vi "RT Main.vi"() -> ()   [LabVIEW 2016]
doc: "This template is for the Queued Message Handler design pattern.\n\nThe Event Handling Loop generates messages based on user interface actions.\n\nThe Message Handling Loop processes messages generated by the Event Handling Loop, or by other messages. The messages are string values, so new messages can be added easily to the Message Cases case structure in the Message Handling Loop. Each message cluster can also provide an optional value for Message Data, which is a variant that can be converted to whatever message-specific data is required."
uses:
  Globale Variablen VI/Global Variables.vi
  Globale Variablen VI/AutonomousMode.vi
  <vilib>/FPGAPlugInAG/cRIO-9067/niLvFpga_Open_cRIO-9067.vi
  <vilib>/rvi/interface/common/dynamic/niFpgaDynamicAddResources.vi
  <vilib>/FPGAPlugInAG/Dynamic/niLvFpga_Run_Dynamic.vi
  <vilib>/Utility/error.llb/Error Cluster From Error Code.vi
  <vilib>/rvi/errors/niLvFpgaAdjustHostInterfaceError.vi
  <vilib>/rvi/interface/nirviOpenFPGA/nirviOpenFPGA.xnode
  FPGA Bitfiles/SUPERFINAL4.0_FPGATarget_CountingFPGA_e4Zp8abhcd8.lvbitx
  FPGA VI/CountingFPGA.vi
  <vilib>/rvi/interface/nirviMethod/nirviMethod.xnode
  <vilib>/rvi/interface/nirviReadWriteControl/nirviReadWriteControl.xnode
  NiFpgaLv.dll
  <vilib>/rvi/interface/Simulation/niFpgaSimulationCallBeginRW.vi
panel:
  out "error out":errorcluster
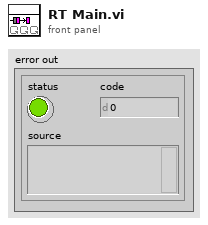
[diagram p1: front panel]
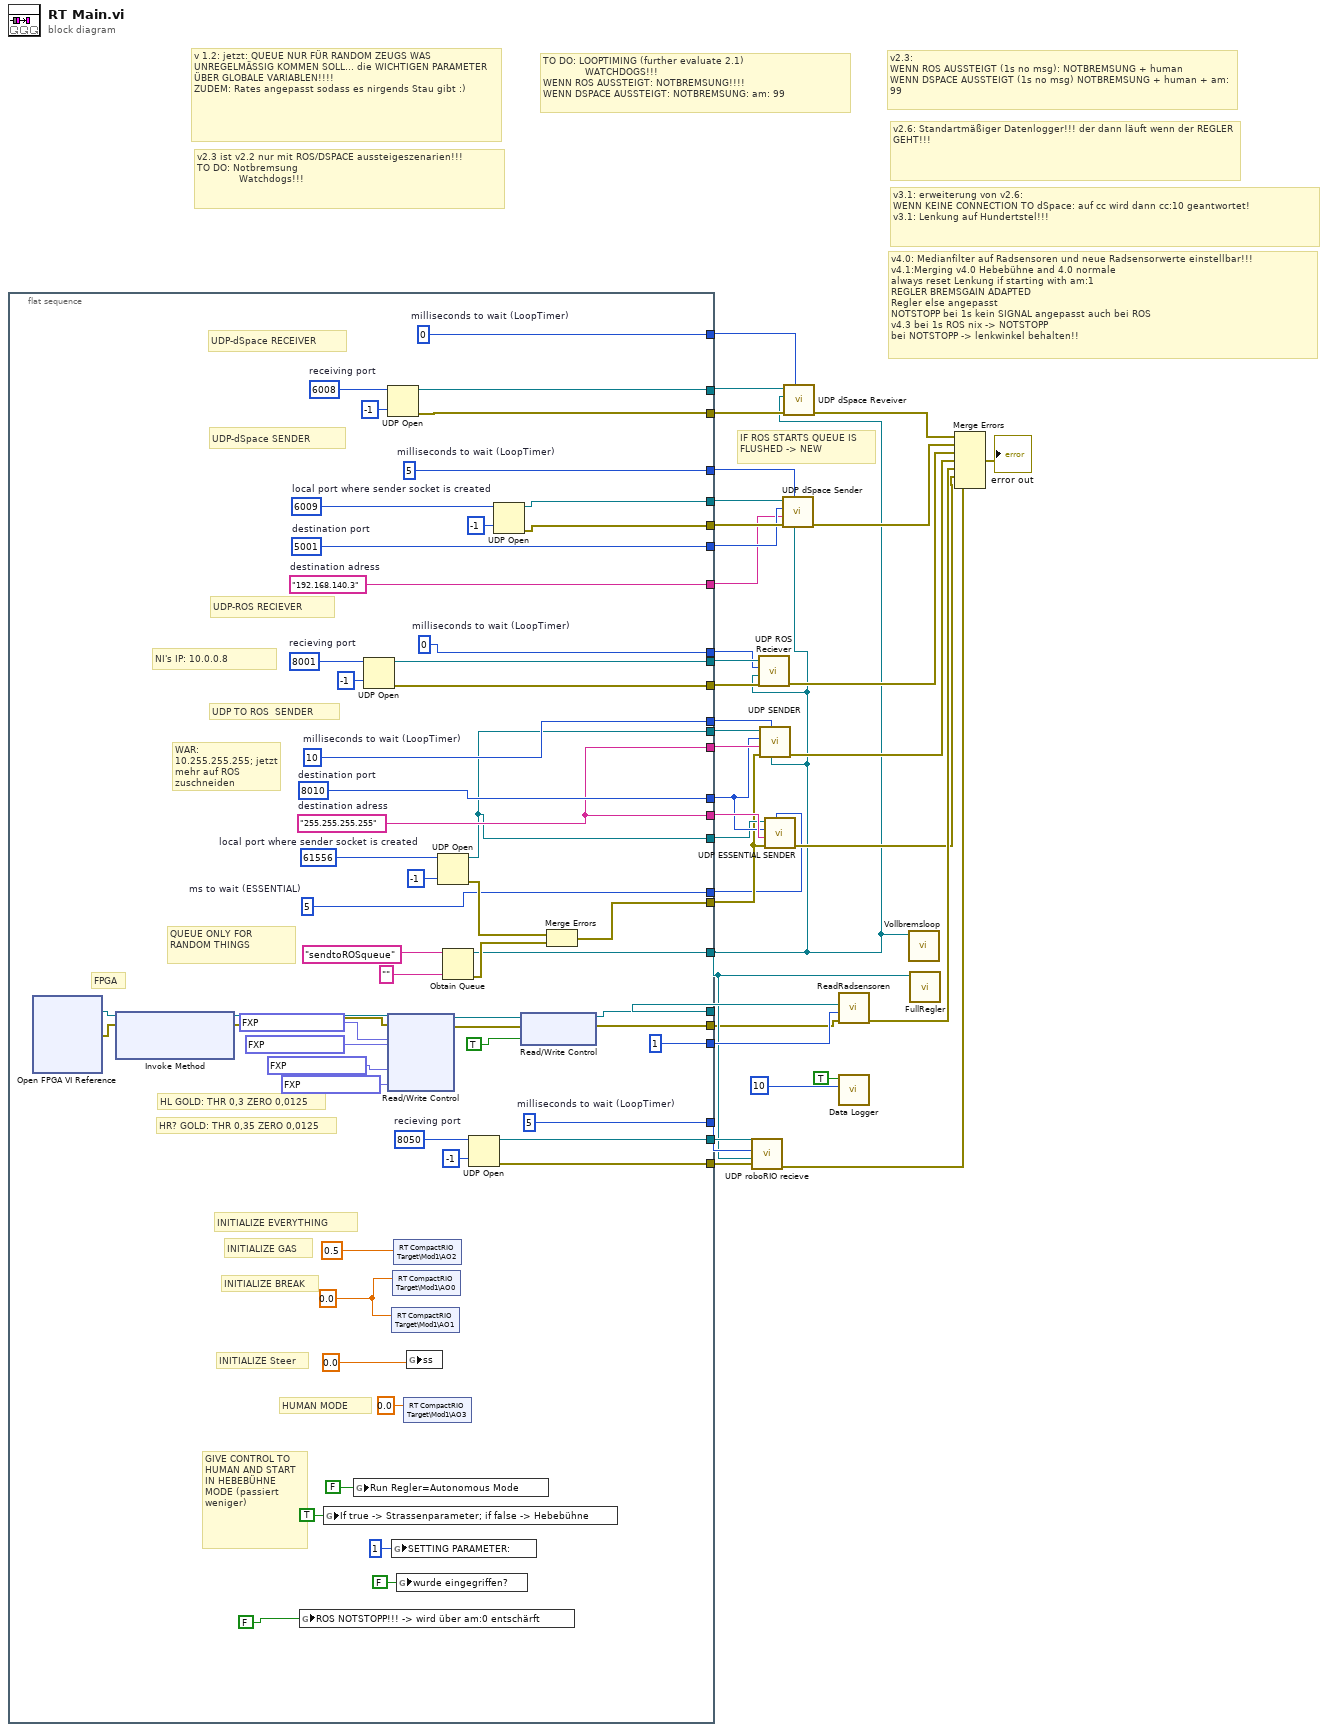
[diagram p0: block diagram]
diagram:
  # "v4.0: Medianfilter auf Radsensoren und neue Radsensorwerte einstellbar!!!\nv4.1:Merging v4.0 Hebebühne and 4.0 normale\nalways reset Lenkung if starting with am:1\nREGLER BREMSGAIN ADAPTED\nRegler else angepasst\nNOTSTOPP bei 1s kein SIGNAL angepasst auch bei ROS\nv4.3 bei 1s ROS nix -> NOTSTOPP\nbei NOTSTOPP -> lenkwinkel behalten!!"
  # "v3.1: erweiterung von v2.6:\nWENN KEINE CONNECTION TO dSpace: auf cc wird dann cc:10 geantwortet!\nv3.1: Lenkung auf Hundertstel!!!"
  # "v2.6: Standartmäßiger Datenlogger!!! der dann läuft wenn der REGLER GEHT!!!"
  # "v2.3:\nWENN ROS AUSSTEIGT (1s no msg): NOTBREMSUNG + human\nWENN DSPACE AUSSTEIGT (1s no msg) NOTBREMSUNG + human + am: 99"
  # "TO DO: LOOPTIMING (further evaluate 2.1)\n              WATCHDOGS!!!\nWENN ROS AUSSTEIGT: NOTBREMSUNG!!!!\nWENN DSPACE AUSSTEIGT: NOTBREMSUNG: am: 99"
  # "v2.3 ist v2.2 nur mit ROS/DSPACE aussteigeszenarien!!!\nTO DO: Notbremsung\n              Watchdogs!!!"
  # "IF ROS STARTS QUEUE IS FLUSHED -> NEW"
  # "v 1.2: jetzt: QUEUE NUR FÜR RANDOM ZEUGS WAS UNREGELMÄSSIG KOMMEN SOLL... die WICHTIGEN PARAMETER ÜBER GLOBALE VARIABLEN!!!!\nZUDEM: Rates angepasst sodass es nirgends Stau gibt :)"
  n1 = flat-sequence {
    tunnel: [w85] -> w36
    tunnel: [w84] -> w35
    tunnel: [w83] -> w34
    tunnel: [w82] -> w33
    tunnel: [w81] -> w32
    tunnel: [w80] -> w31
    tunnel: [w79] -> w30
    tunnel: [w78] -> w29
    tunnel: [w59] -> w28
    tunnel: [w73] -> w12
    tunnel: [w77] -> w27
    tunnel: [w76] -> w14
    tunnel: [w60] -> w26
    tunnel: [w72] -> w20
    tunnel: [w71] -> w19
    tunnel: [w70] -> w18
    tunnel: [u32 1 ("milliseconds to wait")] -> w17
    tunnel: [w61] -> w3
    tunnel: [w38] -> w16
    tunnel: [w60] -> w15
    tunnel: [w59] -> w13
    tunnel: [w58] -> w9
    tunnel: [w52] -> w5
    tunnel: [w51] -> w4
    tunnel: [w50] -> w6
    tunnel: [w37] -> w1
    frame #0 {
      w50 = u32 5  # milliseconds to wait (LoopTimer)
      w54 = u16 8050  # recieving port
      w58 = u32 5  # ms to wait (ESSENTIAL)
      w70 = u32 0  # milliseconds to wait (LoopTimer)
      w71 = u32 5  # milliseconds to wait (LoopTimer)
      w72 = u32 0  # milliseconds to wait (LoopTimer)
      w77 = u32 10  # milliseconds to wait (LoopTimer)
      w76 = u16 8010  # destination port
      w88 = u16 61556  # local port where sender socket is created
      w60 = "255.255.255.255"  # destination adress
      w90 = 0.0
      w92 = u16 8001  # recieving port
      w81 = u16 5001  # destination port
      w93 = u16 6009  # local port where sender socket is created
      w80 = "192.168.140.3"  # destination adress
      w94 = u16 6008  # receiving port
      # "HR? GOLD: THR 0,35 ZERO 0,0125"
      # "HL GOLD: THR 0,3 ZERO 0,0125"
      # "HUMAN MODE"
      # "WAR: 10.255.255.255; jetzt mehr auf ROS zuschneiden"
      # "NI's IP: 10.0.0.8"
      # "GIVE CONTROL TO   HUMAN AND START IN HEBEBÜHNE MODE (passiert weniger)"
      # "INITIALIZE EVERYTHING"
      # "QUEUE ONLY FOR RANDOM THINGS"
      # "FPGA"
      # "UDP TO ROS  SENDER"
      # "INITIALIZE Steer"
      # "INITIALIZE BREAK"
      # "INITIALIZE GAS"
      # "UDP-ROS RECIEVER"
      # "UDP-dSpace SENDER"
      # "UDP-dSpace RECEIVER"
      n2 = xnode "Open FPGA VI Reference"() -> ("FPGA VI Reference Out"=w49:refnum<k20>, "error out"=w48:errorcluster)  [unwired: 2 in]
      n3 = xnode "Invoke Method"("FPGA VI Reference In"=w49, "error in"=w48) -> ("FPGA VI Reference Out"=w43:refnum<k20>, "error out"=w42:errorcluster)  [unwired: 1 in]
      n4 = global write "AutonomousMode.vi" "ROS NOTSTOPP!!! -> wird über am:0 entschärft"(FALSE ("wurde eingegriffen?")) -> ()
      n5 = global write "AutonomousMode.vi" "If true -> Strassenparameter; if false -> Hebebühne"(TRUE ("If true -> Strassenparameter; if false -> Hebebühne")) -> ()
      n6 = global write "AutonomousMode.vi" "Run Regler=Autonomous Mode"(FALSE ("Autonomous Mode")) -> ()
      n7 = UDP Open(9:-1 ("timeout ms (25000)"), 11:w92) -> (port=w79:refnum<k16>, 0:w78:errorcluster)  [unwired: 3 in, 1 out]
      n8 = UDP Open(9:-1 ("timeout ms (25000)"), 11:w94) -> (port=w85:refnum<k16>, 0:w84:errorcluster)  [unwired: 3 in, 1 out]
      n9 = xnode "Read/Write Control"("FPGA VI Reference In"=w43, "error in"=w42, "THR HR"=fxp<+,18,3> 0.350006103515625, "ZERO HR"=fxp<+,18,3> 0.01251220703125, "THR HL"=fxp<+,18,3> 0.29998779296875, "ZERO HL"=fxp<+,18,3> 0.01251220703125) -> ("FPGA VI Reference Out"=w41:refnum<k20>, "error out"=w40:errorcluster)
      n10 = shared-variable "RT CompactRIO Target\\Mod1\\AO1"(w90) -> ()  [unwired: 1 in, 1 out]
      n11 = global write "Global Variables.vi" "SETTING PARAMETER:"(1 ("SETTING PARAMETER:\n0: DO NOTHING\n1: SET TO HUMAN MODE\n2: ENABLE REGLER")) -> ()
      n12 = shared-variable "RT CompactRIO Target\\Mod1\\AO0"(w90) -> ()  [unwired: 1 in, 1 out]
      n13 = shared-variable "RT CompactRIO Target\\Mod1\\AO2"(0.5) -> ()  [unwired: 1 in, 1 out]
      n14 = global write "Global Variables.vi" "wurde eingegriffen?"(FALSE ("wurde eingegriffen?")) -> ()
      n15 = shared-variable "RT CompactRIO Target\\Mod1\\AO3"(0.0 ("AO3")) -> ()  [unwired: 1 in, 1 out]
      n16 = global write "Global Variables.vi" "ss"(0.0 ("ss")) -> ()
      n17 = UDP Open(9:-1 ("timeout ms (25000)"), 11:w88) -> (port=w59:refnum<k16>, 0:w74:errorcluster)  [unwired: 3 in, 1 out]
      n18 = Obtain Queue(name (unnamed)="sendtoROSqueue", element data type="") -> (queue out=w61:refnum<queue>, error out=w75:errorcluster)  [unwired: 3 in, 1 out]
      n19 = UDP Open(9:-1 ("timeout ms (25000)"), 11:w54) -> (port=w52:refnum<k16>, 0:w51:errorcluster)  [unwired: 3 in, 1 out]
      n20 = UDP Open(9:-1 ("timeout ms (25000)"), 11:w93) -> (port=w83:refnum<k16>, 0:w82:errorcluster)  [unwired: 3 in, 1 out]
      n21 = xnode "Read/Write Control"("FPGA VI Reference In"=w41, "error in"=w40, "stop if true"=TRUE) -> ("FPGA VI Reference Out"=w38:refnum<k20>, "error out"=w37:errorcluster)
      n22 = Merge Errors(w74, w75) -> (w73:errorcluster)
    }
  }
  n23 = call "UDP roboRIO recieve.vi"("error in (no error)"=w4, "ENQUE DIRECTLY"=w3, "milliseconds to wait"=w6, "UDP Network Connection in"=w5) -> ("error out"=w2:errorcluster)  [unwired: 7 in]
  n24 = call "UDP ROS Reciever.vi"("error in (no error)"=w29, "ENQUE DIRECTLY"=w3, "milliseconds to wait"=w20, "UDP Network Connection in"=w30) -> ("error out"=w23:errorcluster)  [unwired: 7 in]
  n25 = call "UDP SENDER.vi"("queue"=w3, "milliseconds to wait (LoopTimer)"=w27, "error in (no error)"=w12, "destination adress"=w26, "destination port"=w14, "UDP Network Connection in"=w28) -> ("error out"=w22:errorcluster)  [unwired: 5 in]
  n26 = call "UDP ESSENTIAL SENDER.vi"("milliseconds to wait (LoopTimer)"=w9, "error in (no error)"=w12, "destination adress"=w15, "destination port"=w14, "UDP Network Connection in"=w13) -> ("error out"=w10:errorcluster)  [unwired: 6 in]
  n27 = call "UDP dSpace Sender.vi"("ENQUE DIRECTLY"=w3, "milliseconds to wait"=w19, "error in (no error)"=w33, "destination adress"=w31, "destination port"=w32, "UDP Network Connection in"=w34) -> ("error out"=w24:errorcluster)  [unwired: 5 in]
  n28 = call "UDP dSpace Reveiver.vi"("milliseconds to wait"=w18, "error in (no error)"=w35, "ENQUE DIRECTLY"=w3, "UDP Network Connection in"=w36) -> ("error out"=w25:errorcluster)  [unwired: 7 in]
  n29 = call "ReadRadsensoren.vi"("error in (no error)"=w1, "milliseconds to wait"=w17, "FPGA VI Reference Out"=w16) -> ("error out"=w11:errorcluster)  [unwired: 8 in]
  n30 = call "Data Logger.vi"("logging rate (ms)"=u32 10, "YOU WANT TO LOG?"=TRUE) -> ()  [unwired: 10 in]
  n31 = call "Vollbremsloop.vi"("Queue in"=w3) -> ()  [unwired: 11 in]
  n32 = call "FullRegler.vi"("Queue in"=w3) -> ()  [unwired: 11 in]
  n33 = Merge Errors(w25, w24, w23, w22, w11, w10, w2) -> (→"error out":errorcluster)
